vi "Atto DRY Interface get Cryostat Out Pressure.vi"(8 "error in (no error)":errorcluster, 11 "CryostatOutPressureMbar":sgl) -> (0 "error out":errorcluster, 2 "function return":i32, 3 "CryostatOutPressureMbar out":sgl)   [LabVIEW 2016, in "attoDRYLib.lvlib"]
doc: "int32_t __cdecl AttoDRY_Interface_getCryostatOutPressure(\n float *CryostatOutPressureMbar);"
uses:
  <userlib>/attoDRYLib/attoDRYLib.lvlib
  <userlib>/attoDRYLib/attoDRYLib.dll
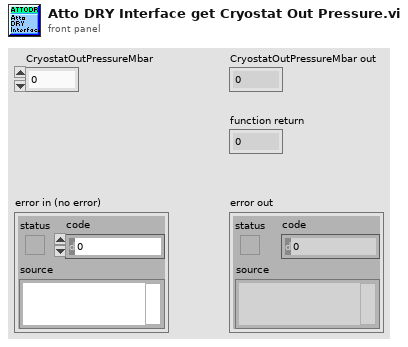
[diagram p1: front panel]
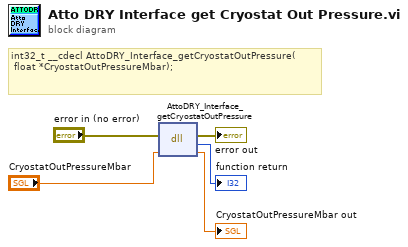
[diagram p0: block diagram]
diagram:
  # "int32_t __cdecl AttoDRY_Interface_getCryostatOutPressure(\n\tfloat *CryostatOutPressureMbar);"
  n1 = dll-call lib="C:/Program Files (x86)/National Instruments/LabVIEW 2016/user.lib/attoDRYLib/attoDRYLib.*" fn="AttoDRY_Interface_getCryostatOutPressure"(error in="error in (no error)", "CryostatOutPressureMbar"="CryostatOutPressureMbar") -> (error out=→"error out":errorcluster, →"function return":i32, "CryostatOutPressureMbar"=→"CryostatOutPressureMbar out":sgl)  [unwired: 2 in, 1 out]
